vi "State Machine-JDS.vi"() -> ()   [LabVIEW 2014]
doc: "This VI is a template for a state machine. Just replace Process 1 and Process 2 with your states. To add more processes, modify the type defined enumerated constant. Enum order must match cluster order."
panel:
  in  "stop":bool
  in  "Process 2":bool
  in  "Process 1":bool
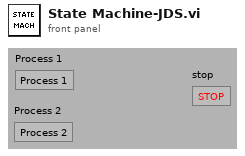
[diagram p1: front panel]
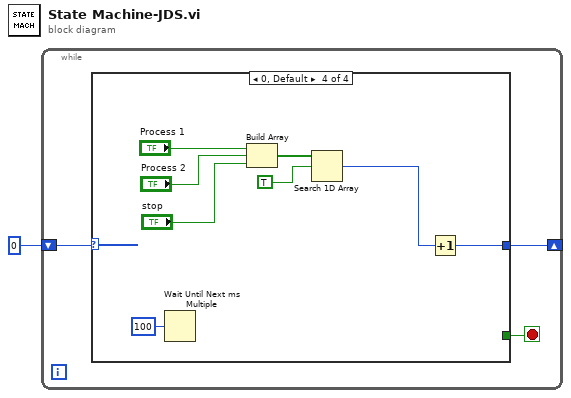
[diagram p0: block diagram]
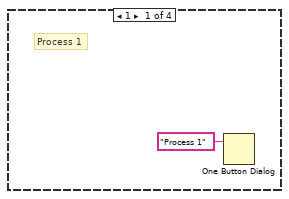
[diagram p2: hidden frame]
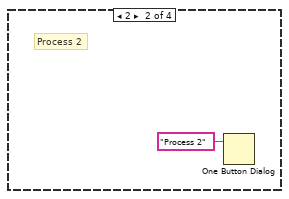
[diagram p3: hidden frame]
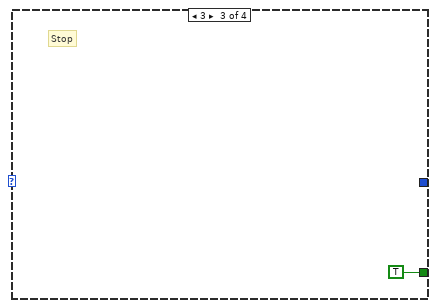
[diagram p4: hidden frame]
diagram:
  n1 = while {
    shift-right: [w3] -> _
    shift-left: 0 -> [w4]
    stop <- w2 stop-if-true
    n2 = case shown="0, Default" w4 {
      tunnel: [_ _ _ w8] -> w3
      tunnel: [_ _ TRUE _] -> w2
      frame 1 {
        # "Process 1"
        n3 = One Button Dialog(message="Process 1") -> ()  [unwired: 1 in, 1 out]
      }
      frame 2 {
        # "Process 2"
        n4 = One Button Dialog(message="Process 2") -> ()  [unwired: 1 in, 1 out]
      }
      frame 3 {
        # "Stop"
      }
      frame 0, Default {
        n5 = Wait Until Next ms Multiple(millisecond multiple=u32 100) -> ()  [unwired: 1 out]
        n6 = Build Array("Process 1", "Process 2", "stop") -> (w11:bool[])
        n7 = Search 1D Array(1D array=w11, element=TRUE) -> (index of element=w9:i32)  [unwired: 1 in]
        n8 = Increment(x=w9) -> (x+1=w8:i32)
      }
    }
  }
